vi "Pfeiffer Vacuum HLT5xx Measure.vi"(8 "error in (no error)":errorcluster, 9 "HLT 5xx Measure - Cluster":T1={"Parameter"=5, "Parameter\nread only<->describe"=FALSE, "off<->on"=TRUE, "Trigger 1 in"=1e-09} {"Trigger 1 in" min=1e-09 max=1000.0 step=1e-09 format="%.2e"; "Parameter" items=[" Pressure Gauge (read only)", " Zero", " Measure Standby", " Sniff Flow (read only)", " Leakrate  (read only)", " Leakrate  [mbarl/s] (read only)", " Pressure p1 (read only)", " Pressure p2 (read only)", " Trigger 1", " Gauge Type (read only)", " External Pressure Gauge (read only)"]}, 10 "Adress of unit":u16=1 min=1 max=999 step=1, 11 "COM Port Name in":refnum<visa-resource-name>="COM1") -> (0 "error out":errorcluster, 3 "response (data)":string)   [LabVIEW 2021]
doc: "This VI is an example of how to use the Pfeiffer Vacuum subVIs programmatically. This VI first initializes the instrument, takes measurements, then closes the instrument."
uses:
  <instrlib>/Pfeiffer Vacuum/Public/LeakDetector/PV HLT5xx Measure - Cluster.ctl
  <instrlib>/Pfeiffer Vacuum/Pfeiffer Vacuum.lvlib
panel:
  # "Zero                          :  off  <-------------------> on \n Measure Standby  :  off  <-------------------> on"
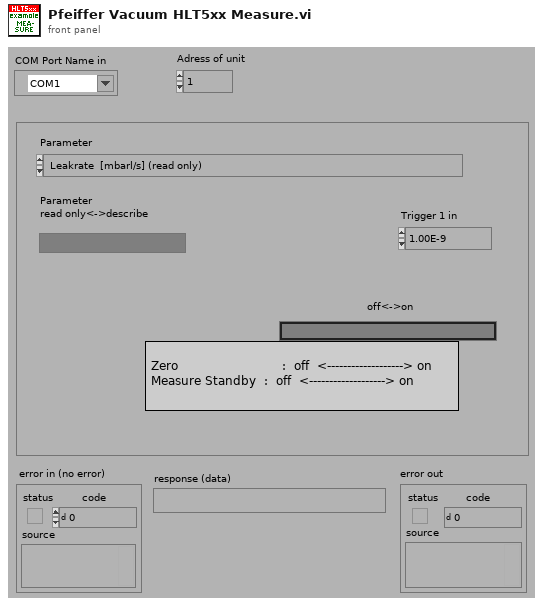
[diagram p1: front panel]
types:
  T1 = typedef "Pfeiffer Vacuum.lvlib/PV HLT5xx Measure - Cluster.ctl" = cluster{"Parameter":u16, "Parameter\nread only<->describe":bool, "off<->on":bool, "Trigger 1 in":dbl}
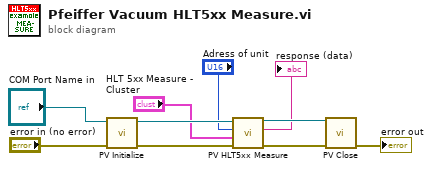
[diagram p0: block diagram]
diagram:
  n1 = call <instrlib>:"PV Initialize.vi"("error in (no error)"="error in (no error)", "VISA session in"="COM Port Name in") -> ("error out"=w10:errorcluster, "VISA session out"=w8:refnum<visa-resource-name>)  [unwired: 8 in]
  n2 = call <instrlib>:"PV HLT5xx Measure.vi"("error in (no error)"=w10, "HLT 5xx Measure - Cluster"="HLT 5xx Measure - Cluster", "Adress of unit"="Adress of unit", "VISA session"=w8) -> ("error out"=w9:errorcluster, "response (data)"=→"response (data)":string, "dup VISA session"=w7:refnum<visa-resource-name>)  [unwired: 5 in]
  n3 = call <instrlib>:"PV Close.vi"("VISA session"=w7, "error in (no error)"=w9) -> ("error out"=→"error out":errorcluster)  [unwired: 13 in]
